vi "UDT_admittanceLibrary_InverseKinematics.vi"() -> (3 "Unit Test Framework Results":T1)   [LabVIEW 2017]
doc: "Use this template to create a user-defined test VI. Define your test requirements and wire the results to the <b>Result (Test)</b> control. Do not modify the <b>Unit Test Framework Results</b> indicator."
uses:
  <vilib>/utf/common/utf_test_result_troll.ctl
  <vilib>/utf/common/utf_test_result.ctl
  <vilib>/utf/common/utf_test_result_failure.ctl
  <vilib>/utf/common/utf_test_comparison_operators.ctl
  <vilib>/utf/common/utf_vi_tag.ctl
  <vilib>/Control Software Solutions Ltd/UTF Helper/SubVIs/UTF Double Equals.vi
  <vilib>/Control Software Solutions Ltd/UTF Helper/Unit Test Helper.lvlib
  RT/Admittance Controller/admittanceControllerLibrary.lvlib
  <vilib>/utf/NI_UnitTestFramework.lvlib
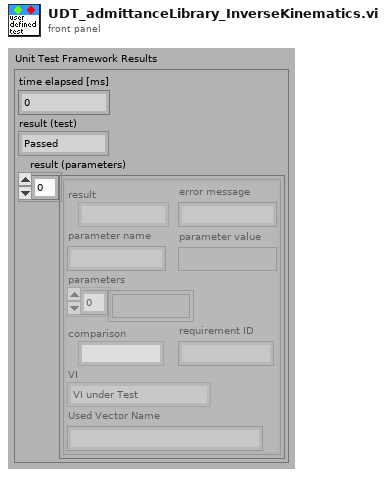
[diagram p1: front panel]
types:
  T1 = typedef "NI_UnitTestFramework.lvlib/utf_test_result_troll.ctl" = cluster{"time elapsed [ms]":u32, "result (test)":T2, "result (parameters)":T3[]}
  T2 = typedef "NI_UnitTestFramework.lvlib/utf_test_result.ctl" = enum16{"Passed", "Failed", "Error", "Skipped", "Not Processed"}
  T3 = typedef "NI_UnitTestFramework.lvlib/utf_test_result_failure.ctl" = cluster{"result":T2, "error message":string, "parameter name":string, "parameter value":variant, "parameters":variant[], "comparison":T4, "requirement ID":string, "VI":T5, "Used Vector Name":string}
  T4 = typedef "NI_UnitTestFramework.lvlib/utf_test_comparison_operators.ctl" = enum16{"=", "!=", ">", ">=", "<", "<=", "range", "symmetric tolerance", "asymmetric tolerance", "string contains", "string not contain", "array size", "string length", "array range", "by element", "array range (limit array)", "user-defined", "array contains", "array not contain", "vector length", "= (elm)", "!= (elm)", "= (case insensitive)", "!= (case insensitive)"}
  T5 = typedef "NI_UnitTestFramework.lvlib/utf_vi_tag.ctl" = enum16{"Setup VI", "VI under Test", "Teardown VI"}
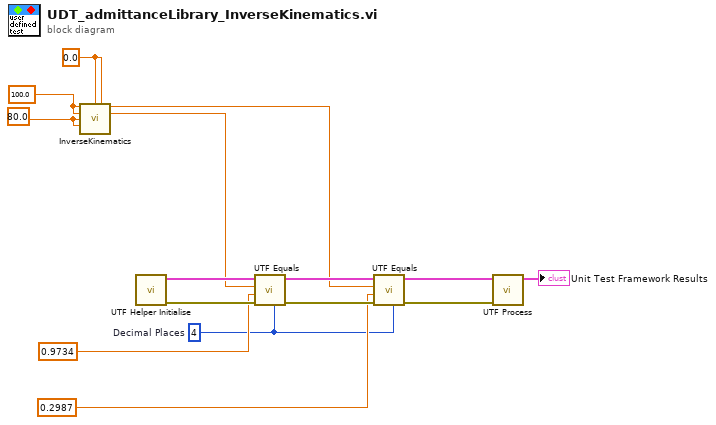
[diagram p0: block diagram]
diagram:
  w1 = u8 4  # Decimal Places
  w4 = 80.0
  w5 = 100.0
  w6 = 0.0
  n1 = call "InverseKinematics.vi"("Next X"=w5, "deltaY"=w6, "deltaX"=w6, "Next Y"=w5, "L0"=w4, "L1"=w4) -> ("destheta0"=w7:dbl, "destheta1"=w8:dbl)  [unwired: 7 in, 1 out]
  n2 = call <vilib>:"UTF Helper Initialise.vi"() -> ("error out"=w9:errorcluster, "results array"=w14:T3[])  [unwired: 10 in]
  n3 = call-poly <vilib>:"UTF Equals.vi"("Decimal Places"=w1, "error in (no error)"=w9, "Test Value"=0.9734, "Input"=w8, "Input Results"=w14) -> ("error out"=w10:errorcluster, "Output Results"=w13:T3[])  [unwired: 5 in]
  n4 = call-poly <vilib>:"UTF Equals.vi"("Decimal Places"=w1, "error in (no error)"=w10, "Test Value"=0.2987, "Input"=w7, "Input Results"=w13) -> ("error out"=w11:errorcluster, "Output Results"=w12:T3[])  [unwired: 5 in]
  n5 = call <vilib>:"UTF Process.vi"("error in (no error)"=w11, "results array"=w12) -> ("Unit Test Framework Results"=→"Unit Test Framework Results":T1)  [unwired: 9 in]
